vi "Format Error Into String.vi"(8 "error in (no error)":errorcluster, 11 "Message Data":variant) -> (0 "error out":errorcluster, 2 "error?":bool, 3 "message":string)   [LabVIEW 2018, in "Personalities Tool.lvlib"]
doc: "This VI formats an incoming error in the Data terminal into a string.\nThis function also clears the error wire."
uses:
  <vilib>/Utility/error.llb/DialogType.ctl
  Personalities Tool.lvlib
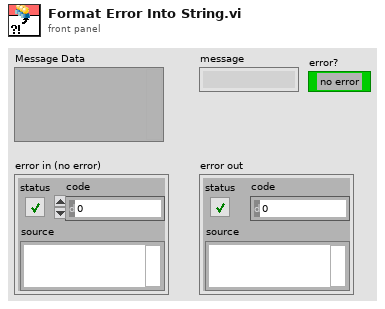
[diagram p1: front panel]
types:
  T1 = typedef "DialogType.ctl" = u16
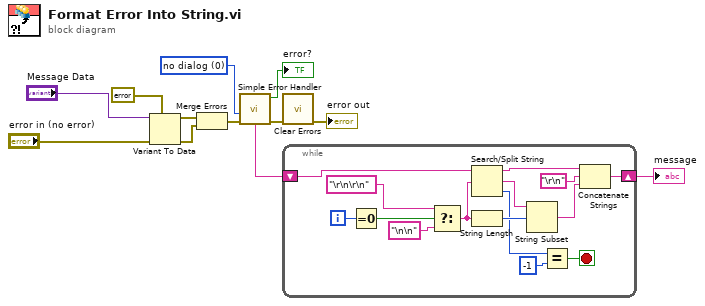
[diagram p0: block diagram]
diagram:
  w10 = T1 0 items=["no dialog", "OK message", "continue or stop message", "OK message + warnings", "continue/stop + warnings"] ("type of dialog (OK msg:1)")
  n1 = Variant To Data(error in="error in (no error)", type=errorcluster {"status"=FALSE, "code"=0, "source"=""} ("error constant"), Variant="Message Data") -> (data=w6:errorcluster, error out=w7:errorcluster)
  n2 = Merge Errors(w6, w7) -> (w9:errorcluster)
  n3 = call <vilib>:"Simple Error Handler.vi"("type of dialog (OK msg:1)"=w10, "error in (no error)"=w9) -> ("error?"=→"error?":bool, "error out"=w2:errorcluster, "message"=w11:string)  [unwired: 3 in, 2 out]
  n4 = call <vilib>:"Clear Errors.vi"("error in (no error)"=w2) -> ("error out"=→"error out":errorcluster)  [unwired: 5 in, 1 out]
  n5 = while {
    shift-right: [w23] -> w12
    shift-left: w11 -> [w27]
    i -> [w17]
    stop <- w19 stop-if-true
    n6 = Equal To 0?(x=w17) -> (x = 0?=w16:bool)
    n7 = Select(t="\r\n\r\n", s=w16, f="\n\n") -> (s? t:f=w13:string)
    n8 = Search/Split String(string=w27, search string/char (-)=w13) -> (substring before match=w22:string, match + rest of string=w26:string, offset of match=w20:i32)  [unwired: 1 in]
    n9 = String Length(string=w13) -> (length=w25:i32)
    n10 = String Subset(string=w26, offset (0)=w25) -> (substring=w24:string)  [unwired: 1 in]
    n11 = Equal?(x=w20, y=-1) -> (x = y?=w19:bool)
    n12 = Concatenate Strings(w22, "\r\n", w24) -> (w23:string)
  }
  "message" <- w12
